vi "Parse Object.vi"(0 "JSON String":string, 5 "Index In":i32, 11 "error in (no error)":errorcluster) -> (4 "Variant out":variant, 6 "Index Out":i32, 15 "error out":errorcluster)   [LabVIEW 2020, in "Variant JSON API.lvlib"]
uses:
  Variant JSON API.lvlib
  Errors.ctl
  Token Type.ctl
  Variant Data Manipulation/Variant Data Manipulation.lvlib
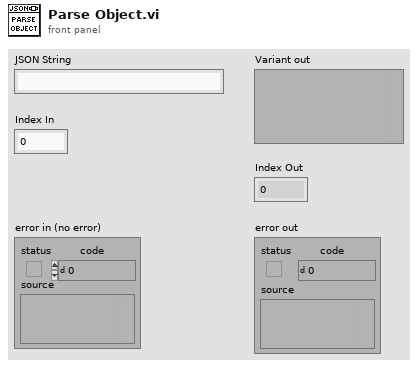
[diagram p1: front panel]
types:
  T1 = typedef "Variant JSON API.lvlib/Errors.ctl" = enum16{"No key", "Key path type", "Array OOB", "Type Mismatch", "Invalid Token", "Invalid Value"}
  T2 = typedef "Variant JSON API.lvlib/Token Type.ctl" = enum16{"NONE", "CURLY_OPEN", "CURLY_CLOSE", "SQUARED_OPEN", "SQUARED_CLOSE", "COLON", "COMMA", "STRING", "NUMBER", "TRUE", "FALSE", "NULL"}
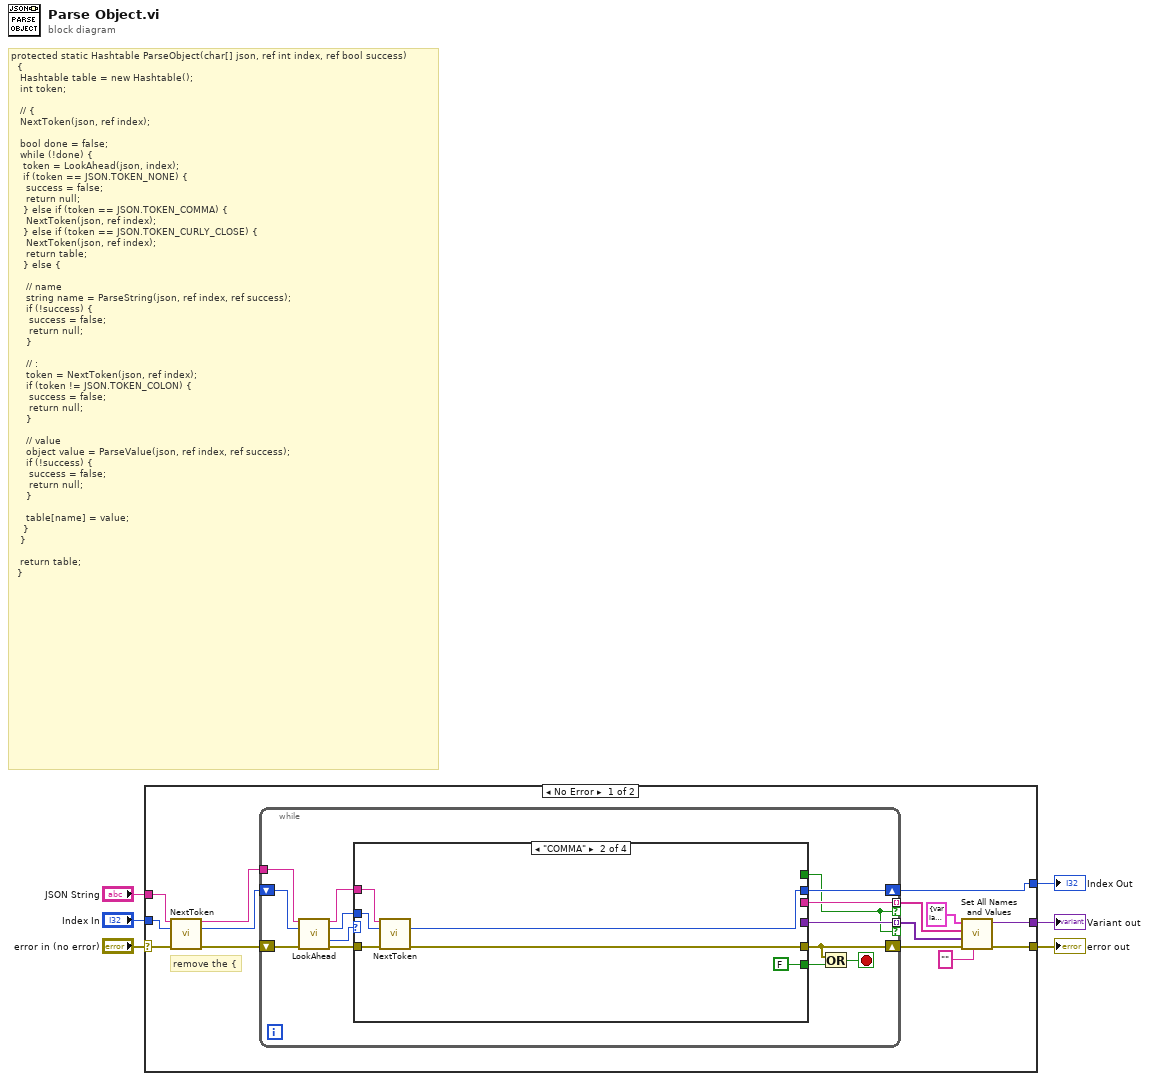
[diagram p0: block diagram]
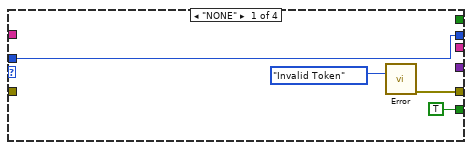
[diagram p2: hidden frame]
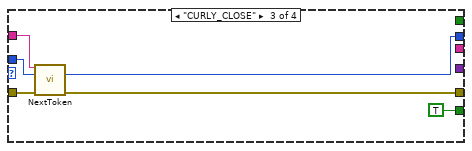
[diagram p3: hidden frame]
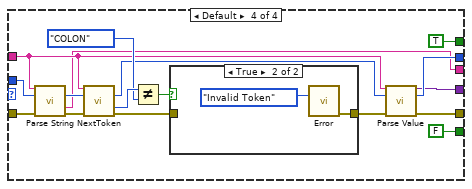
[diagram p4: hidden frame]
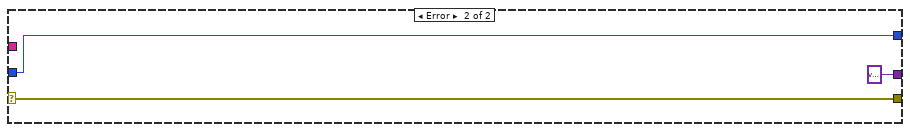
[diagram p6: hidden frame]
diagram:
  # "protected static Hashtable ParseObject(char[] json, ref int index, ref bool success)\n\t\t{\n\t\t\tHashtable table = new Hashtable();\n\t\t\tint token;\n\n\t\t\t// {\n\t\t\tNextToken(json, ref index);\n\n\t\t\tbool done = false;\n\t\t\twhile (!done) {\n\t\t\t\ttoken = LookAhead(json, index);\n\t\t\t\tif (token == JSON.TOKEN_NONE) {\n\t\t\t\t\tsuccess = false;\n\t\t\t\t\treturn null;\n\t\t\t\t} else if (token == JSON.TOKEN_COMMA) {\n\t\t\t\t\tNextToken(json, ref index);\n\t\t\t\t} else if (token == JSON.TOKEN_CURLY_CLOSE) {\n\t\t\t\t\tNextToken(json, ref index);\n\t\t\t\t\treturn table;\n\t\t\t\t} else {\n\n\t\t\t\t\t// name\n\t\t\t\t\tstring name = ParseString(json, ref index, ref success);\n\t\t\t\t\tif (!success) {\n\t\t\t\t\t\tsuccess = false;\n\t\t\t\t\t\treturn null;\n\t\t\t\t\t}\n\n\t\t\t\t\t// :\n\t\t\t\t\ttoken = NextToken(json, ref index);\n\t\t\t\t\tif (token != JSON.TOKEN_COLON) {\n\t\t\t\t\t\tsuccess = false;\n\t\t\t\t\t\treturn null;\n\t\t\t\t\t}\n\n\t\t\t\t\t// value\n\t\t\t\t\tobject value = ParseValue(json, ref index, ref success);\n\t\t\t\t\tif (!success) {\n\t\t\t\t\t\tsuccess = false;\n\t\t\t\t\t\treturn null;\n\t\t\t\t\t}\n\n\t\t\t\t\ttable[name] = value;\n\t\t\t\t}\n\t\t\t}\n\n\t\t\treturn table;\n\t\t}"
  n1 = case shown="No Error" "error in (no error)" {
    selector: "error in (no error)" -> [w16 w72]
    tunnel: [w10 w72] -> w5
    tunnel: "Index In" -> [w17 w73]
    tunnel: [w20 w73] -> w3
    tunnel: [w11 variant ("VCluster")] -> w1
    tunnel: "JSON String" -> [w14 _]
    frame No Error {
      # "remove the {"
      n2 = call "NextToken.vi"("JSON String"=w14, "Index In"=w17, "error in (no error)"=w16) -> ("JSON String Passthrough"=w15:string, "Index Out"=w18:i32, "error out"=w19:errorcluster)  [unwired: 9 in, 1 out]
      n3 = while {
        tunnel: w15 -> [w33]
        shift-right: [w28] -> w20
        shift-left: w18 -> [w32]
        shift-right: [w24] -> w9
        shift-left: w19 -> [w34]
        tunnel: [w23] -> w12 mode=indexing if=w21
        tunnel: [w22] -> w8 mode=indexing if=w21
        stop <- w25 stop-if-true
        n4 = call "LookAhead.vi"("JSON String"=w33, "Index"=w32, "error in (no error)"=w34) -> ("JSON String Passthrough"=w27:string, "Index Passthrough"=w29:i32, "TOKEN"=w31:T2, "error out"=w30:errorcluster)  [unwired: 9 in]
        n5 = case shown="\"COMMA\"" w31 {
          tunnel: [TRUE FALSE TRUE FALSE] -> w26
          tunnel: w30 -> [_ w44 w50 w67]
          tunnel: [w36 w41 w47 w58] -> w24
          tunnel: w29 -> [w37 w43 w49 w66]
          tunnel: [w37 w42 w48 w59] -> w28
          tunnel: w27 -> [_ w39 w45 w61]
          tunnel: [_ _ _ w53] -> w23
          tunnel: [_ _ _ w52] -> w22
          tunnel: [_ _ _ TRUE] -> w21
          frame "NONE" {
            n6 = call "Error.vi"(5:Errors."Invalid Token") -> ("error out"=w36:errorcluster)  [unwired: 14 in]
          }
          frame "COMMA" {
            n7 = call "NextToken.vi"("JSON String"=w39, "Index In"=w43, "error in (no error)"=w44) -> ("Index Out"=w42:i32, "error out"=w41:errorcluster)  [unwired: 9 in, 2 out]
          }
          frame "CURLY_CLOSE" {
            n8 = call "NextToken.vi"("JSON String"=w45, "Index In"=w49, "error in (no error)"=w50) -> ("Index Out"=w48:i32, "error out"=w47:errorcluster)  [unwired: 9 in, 2 out]
          }
          frame Default {
            n9 = call "Parse String.vi"("JSON String"=w61, "Index In"=w66, "error in (no error)"=w67) -> ("Index Out"=w64:i32, "Parsed String"=w53:string, "error out"=w65:errorcluster)  [unwired: 9 in, 1 out]
            n10 = call "NextToken.vi"("JSON String"=w61, "Index In"=w64, "error in (no error)"=w65) -> ("Index Out"=w60:i32, "TOKEN"=w63:T2, "error out"=w54:errorcluster)  [unwired: 9 in, 1 out]
            n11 = Not Equal?(x=w63, y=Token_Type."COLON") -> (x != y?=w56:bool)
            n12 = case shown="True" w56 {
              tunnel: [w68 w69] -> w55
              tunnel: w54 -> [w68 _]
              frame False {
              }
              frame True {
                n13 = call "Error.vi"(5:Errors."Invalid Token") -> ("error out"=w69:errorcluster)  [unwired: 14 in]
              }
            }
            n14 = call "Parse Value.vi"("JSON String"=w61, "Index In"=w60, "error in (no error)"=w55) -> ("Variant out"=w52:variant, "Index Out"=w59:i32, "error out"=w58:errorcluster)  [unwired: 10 in]
          }
        }
        n15 = Or(x=w24, y=w26) -> (x .or. y?=w25:bool)
      }
      n16 = call "Set All Names and Values.vi"("Cluster Name"="" ("Name"), "error in"=w9, "values"=w8, "Element Names"=w12, "Cluster in"=cluster{"Variant out":variant} {"Variant out"=variant}) -> ("error out"=w10:errorcluster, "Cluster out"=w11:variant)  [unwired: 5 in]
    }
    frame Error {
    }
  }
  "error out" <- w5
  "Index Out" <- w3
  "Variant out" <- w1
